vi "Initial Data.vi"(8 "error in (no error)":errorcluster, 11 "Master in":refnum<class "MASTER.lvclass">) -> (0 "error out":errorcluster, 3 "Master out":refnum<class "MASTER.lvclass">)   [LabVIEW 2014, in "Files Library.lvlib" / "Master.lvclass"]
uses:
  MASTER/MASTER.lvclass
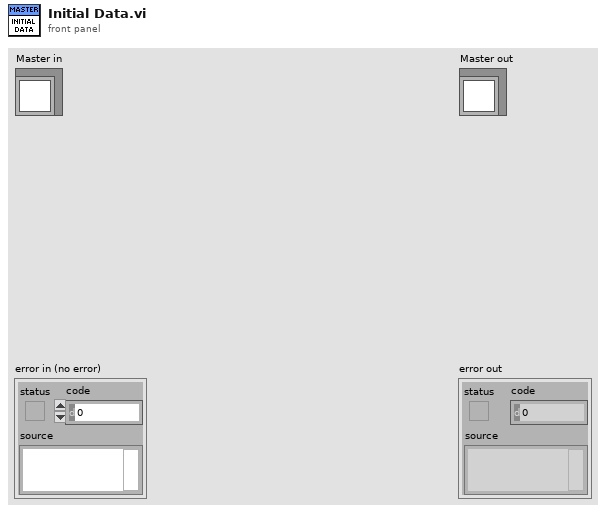
[diagram p1: front panel]
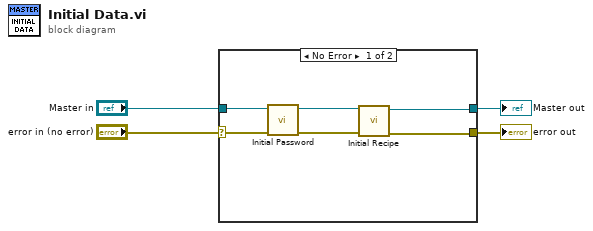
[diagram p0: block diagram]
diagram:
  n1 = case shown="No Error" "error in (no error)" {
    selector: "error in (no error)" -> [w9 w12]
    tunnel: [w5 w12] -> w3
    tunnel: [w6 w11] -> w1
    tunnel: "Master in" -> [w10 w11]
    frame No Error {
      n2 = call-dynamic "Initial Password.vi"("error in (no error)"=w9, "Master in"=w10) -> ("error out"=w7:errorcluster, "Master out"=w8:refnum<class "MASTER.lvclass">)  [unwired: 8 in]
      n3 = call-dynamic "Initial Recipe.vi"("error in (no error)"=w7, "MASTER in"=w8) -> ("error out"=w5:errorcluster, "MASTER out"=w6:refnum<class "MASTER.lvclass">)  [unwired: 8 in]
    }
    frame Error {
    }
  }
  "error out" <- w3
  "Master out" <- w1
